vi "punkt_mit _variabler_größe_zeichnen.vi"(5 "Color":u32(colorbox)=16711680, 6 "x":sgl, 9 "y":sgl, 10 "größe":sgl, 11 "Refnum in":T1) -> (0 "output cluster":cluster{sgl, sgl, sgl, sgl}, 3 "Refnum out":T1)   [LabVIEW 2014]
uses:
  <vilib>/vision/Image Controls.llb/IMAQ Image.ctl
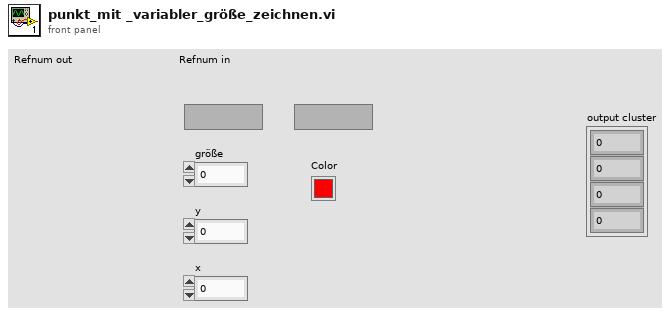
[diagram p1: front panel]
types:
  T1 = typedef "IMAQ Image.ctl" = refnum<image>
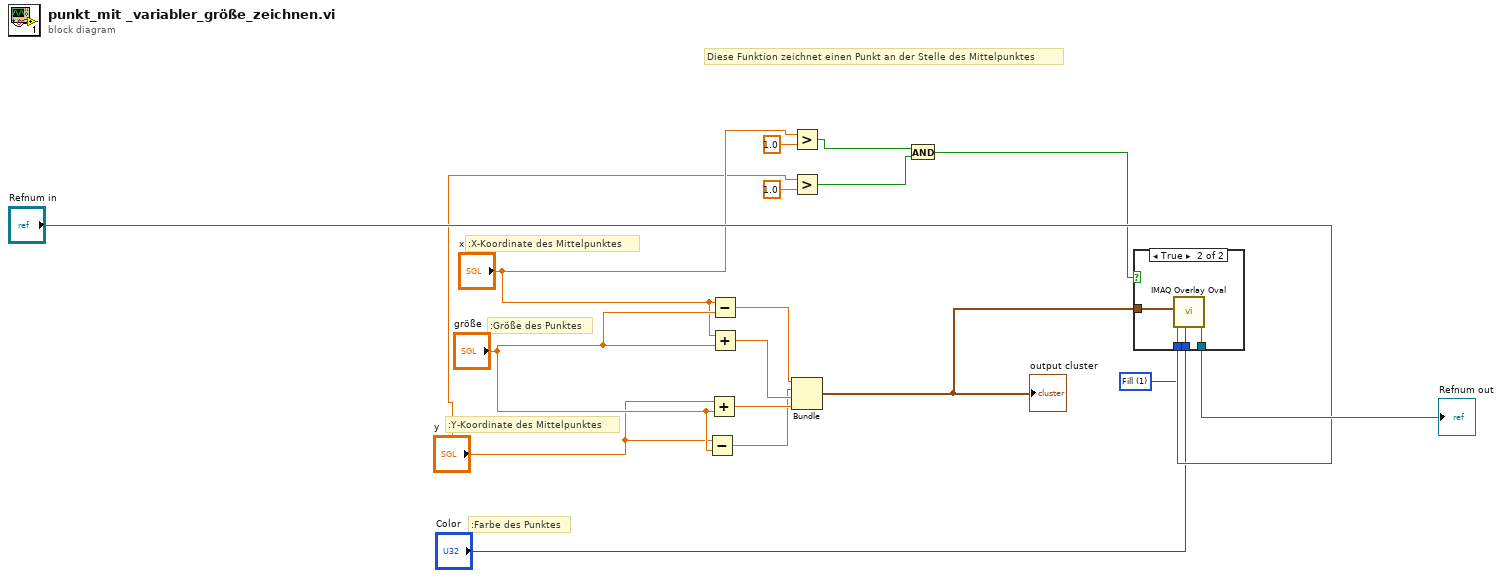
[diagram p0: block diagram]
diagram:
  w14 = u32 1 items=["Frame", "Fill"] ("Drawing Mode (Frame)")
  # ":Farbe des Punktes"
  # ":Größe des Punktes"
  # ":Y-Koordinate des Mittelpunktes"
  # ":X-Koordinate des Mittelpunktes"
  # "Diese Funktion zeichnet einen Punkt an der Stelle des Mittelpunktes"
  n1 = Subtract(x="y", y="größe") -> (x-y=w10:sgl)
  n2 = Add(x="y", y="größe") -> (x+y=w12:sgl)
  n3 = Subtract(x="x", y="größe") -> (x-y=w9:sgl)
  n4 = Add(x="x", y="größe") -> (x+y=w11:sgl)
  n5 = Greater?(x="x", y=sgl 1.0) -> (0:w5:bool)
  n6 = Greater?(x="y", y=sgl 1.0) -> (0:w4:bool)
  n7 = Bundle(w9, w10, w11, w12) -> (w13:cluster{sgl, sgl, sgl, sgl})  [unwired: 1 in]
  "output cluster" <- w13
  n8 = And(x=w5, y=w4) -> (x .and. y?=w3:bool)
  n9 = case shown="True" w3 {
    tunnel: [w18 w23] -> w16
    tunnel: "Refnum in" -> [w18 w22]
    tunnel: w14 -> [_ w21]
    tunnel: w13 -> [_ w20]
    tunnel: "Color" -> [_ w19]
    frame False {
    }
    frame True {
      n10 = call "IMAQ Overlay Oval"("Color"=w19, "Drawing Mode (Frame)"=w21, "Bounding Rectangle"=w20, "Image"=w22) -> ("Image Out"=w23:T1)  [unwired: 6 in, 1 out]
    }
  }
  "Refnum out" <- w16
